vi "Construct Connection Factory Handler.vi"(10 "Log Instance":refnum<class "LoggerReference.lvclass">, 11 "Connection Factory Type":refnum<class "IConnectionFactory.lvclass">) -> (3 "ConnectionFactoryHandler":refnum<class "ConnectionFactoryHandler.lvclass">)   [LabVIEW 2020, in "ConnectionFactorySession.lvlib" / "ConnectionFactoryHandler.lvclass"]
uses:
  <vilib>/gpm_packages/@cs/Network-interface/Source/Connection Factory Session/ConnectionFactoryHandler/ConnectionFactoryHandler.lvclass
  C:/Program Files/National Instruments/LabVIEW 2020/vi.lib/gpm_packages/@cs/Network-interface/Source/Logged Actor/LoggedActor.lvclass
  <vilib>/gpm_packages/@cs/Network-interface/Source/IConnectionFactory/IConnectionFactory.lvclass
  <vilib>/gpm_packages/@cs/event-logger/Source/Composed Log/LoggerReference/LoggerReference.lvclass
  <vilib>/gpm_packages/@cs/Network-interface/Source/Connection Factory Session/ConnectionFactoryHandler/ConnectionFactoryHandler.lvclass/ConnectionFactoryHandler.ctl
  <vilib>/gpm_packages/@cs/Network-interface/Source/Logged Actor/LoggedActor.lvclass/LoggedActor.ctl
  <vilib>/gpm_packages/@cs/Network-interface/Source/Logged Actor/LoggedActor.lvclass
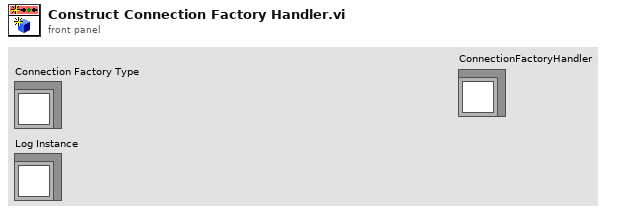
[diagram p1: front panel]
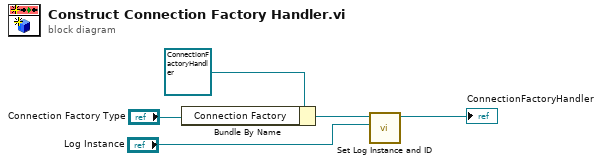
[diagram p0: block diagram]
diagram:
  n1 = Bundle By Name(cluster=refnum<class "ConnectionFactoryHandler.lvclass"> refnum ("ConnectionFactoryHandler in"), "Connection Factory"="Connection Factory Type") -> (w3:refnum<class "ConnectionFactoryHandler.lvclass">)
  n2 = call <vilib>:"Set Log Instance and ID.vi"("Log Instance"="Log Instance", "LoggedActor in"=w3) -> ("LoggedActor out"=→"ConnectionFactoryHandler":refnum<class "ConnectionFactoryHandler.lvclass">)  [unwired: 9 in]
